vi "Exit.vi"(6 "Priority (F)":bool, 7 "Process Name":string, 8 "error in (no error)":errorcluster) -> (0 "error out":errorcluster)   [LabVIEW 2016, in "System.lvlib"]
uses:
  System.lvlib
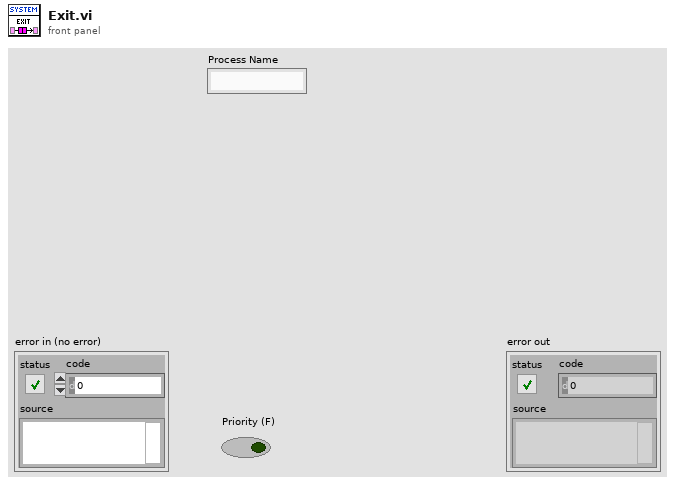
[diagram p1: front panel]
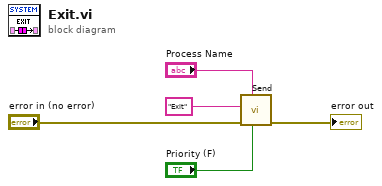
[diagram p0: block diagram]
diagram:
  n1 = call "Send.vi"("Priority (F)"="Priority (F)", "Process Name"="Process Name", "error in (no error)"="error in (no error)", "Message"="Exit") -> ("error out"=→"error out":errorcluster)  [unwired: 7 in]
